vi "fp display engine resonance.vi"(7 "channel data in":sgl[][][](array[numeric]), 10 "Image Refs In":T1[](array[typedef]), 11 "DisplayRefsIn(generic class)":refnum<vi>[](array[refnum])) -> ()   [LabVIEW 2012]
uses:
  <vilib>/vision/Image Controls.llb/IMAQ Image.ctl
  Custom Controls/Ch selector.ctl
  GFG/GFGfpRefGet.vi
  GFG/GFGbooleanGet.vi
  Custom Controls/MAIN Image panel tab Control type def.ctl
  <vilib>/vision/NI_Vision_Development_Module.lvlib
  GFG/GFG library.lvlib
panel:
  in  "ROI colors":u32[](array[colorbox])=[6618880, 16716362, 16860, 16776793, 16750848, 16448250, 16716530, 9567230, 16764108, 7340212, 32639, 0, 13816530, 8421376, 8421631, 7171459, 6618880, 16716362, 16860, 16776793, 16750848, 16448250, 16716530, 9567230, 16764108, 7340212, 32639, 0, 13816530, 8421376, 8421631, 7171459, 6618880, 16716362, 16860, 16776793, 16750848, 16448250, 16716530, 9567230, 16764108, 7340212, 32639, 0, 13816530, 8421376, 8421631, 7171459, 6618880, 16716362, 16860, 16776793, 16750848, 16448250, 16716530, 9567230, 16764108, 7340212, 32639, 0, 13816530, 8421376, 8421631, 7171459, 6618880, 16716362, 16860, 16776793, 16750848, 16448250, 16716530, 9567230, 16764108, 7340212, 32639, 0, 13816530, 8421376, 8421631, 7171459, 6618880, 16716362, 16860, 16776793, 16750848, 16448250, 16716530, 9567230, 16764108, 7340212, 32639, 0, 13816530, 8421376, 8421631, 7171459, 6618880, 16716362, 16860, 16776793, 16750848, 16448250, 16716530, 9567230, 16764108, 7340212, 32639, 0, 13816530, 8421376, 8421631, 7171459, 6618880, 16716362, 16860, 16776793, 16750848, 16448250, 16716530, 9567230, 16764108, 7340212, 32639, 0, 13816530, 8421376, 8421631, 7171459, 6618880, 16716362, 16860, 16776793, 16750848, 16448250, 16716530, 9567230, 16764108, 7340212, 32639, 0, 13816530, 8421376, 8421631, 7171459, 6618880, 16716362, 16860, 16776793, 16750848, 16448250, 16716530, 9567230, 16764108, 7340212, 32639, 0, 13816530, 8421376, 8421631, 7171459, 6618880, 16716362, 16860, 16776793, 16750848, 16448250, 16716530, 9567230, 16764108, 7340212, 32639, 0, 13816530, 8421376, 8421631, 7171459, 6618880, 16716362, 16860, 16776793, 16750848, 16448250, 16716530, 9567230, 16764108, 7340212, 32639, 0, 13816530, 8421376, 8421631, 7171459, 6618880, 16716362, 16860, 16776793, 16750848, 16448250, 16716530, 9567230, 16764108, 7340212, 32639, 0, 13816530, 8421376, 8421631, 7171459, 6618880, 16716362, 16860, 16776793, 16750848, 16448250, 16716530, 9567230, 16764108, 7340212, 32639, 0, 13816530, 8421376, 8421631, 7171459, 6618880, 16716362, 16860, 16776793, 16750848, 16448250, 16716530, 9567230, 16764108, 7340212, 32639, 0, 13816530, 8421376, 8421631, 7171459, 6618880, 16716362, 16860, 16776793, 16750848, 16448250, 16716530, 9567230, 16764108, 7340212, 32639, 0, 13816530, 8421376, 8421631, 7171459, 6618880, 16716362, 16860, 16776793, 16750848, 16448250, 16716530, 9567230, 16764108, 7340212, 32639, 0, 13816530, 8421376, 8421631, 7171459, 6618880, 16716362, 16860, 16776793, 16750848, 16448250, 16716530, 9567230, 16764108, 7340212, 32639, 0, 13816530, 8421376, 8421631, 7171459, 6618880, 16716362, 16860, 16776793, 16750848, 16448250, 16716530, 9567230, 16764108, 7340212, 32639, 0, 13816530, 8421376, 8421631, 7171459, 6618880, 16716362, 16860, 16776793, 16750848, 16448250, 16716530, 9567230, 16764108, 7340212, 32639, 0, 13816530, 8421376, 8421631, 7171459, 6618880, 16716362, 16860, 16776793, 16750848, 16448250, 16716530, 9567230, 16764108, 7340212, 32639, 0, 13816530, 8421376, 8421631, 7171459, 6618880, 16716362, 16860, 16776793, 16750848, 16448250, 16716530, 9567230, 16764108, 7340212, 32639, 0, 13816530, 8421376, 8421631, 7171459, 6618880, 16716362, 16860, 16776793, 16750848, 16448250, 16716530, 9567230, 16764108, 7340212, 32639, 0, 13816530, 8421376, 8421631, 7171459, 6618880, 16716362, 16860, 16776793, 16750848, 16448250, 16716530, 9567230, 16764108, 7340212, 32639, 0, 13816530, 8421376, 8421631, 7171459, 6618880, 16716362, 16860, 16776793, 16750848, 16448250, 16716530, 9567230, 16764108, 7340212, 32639, 0, 13816530, 8421376, 8421631, 7171459]
  out "error out":errorcluster
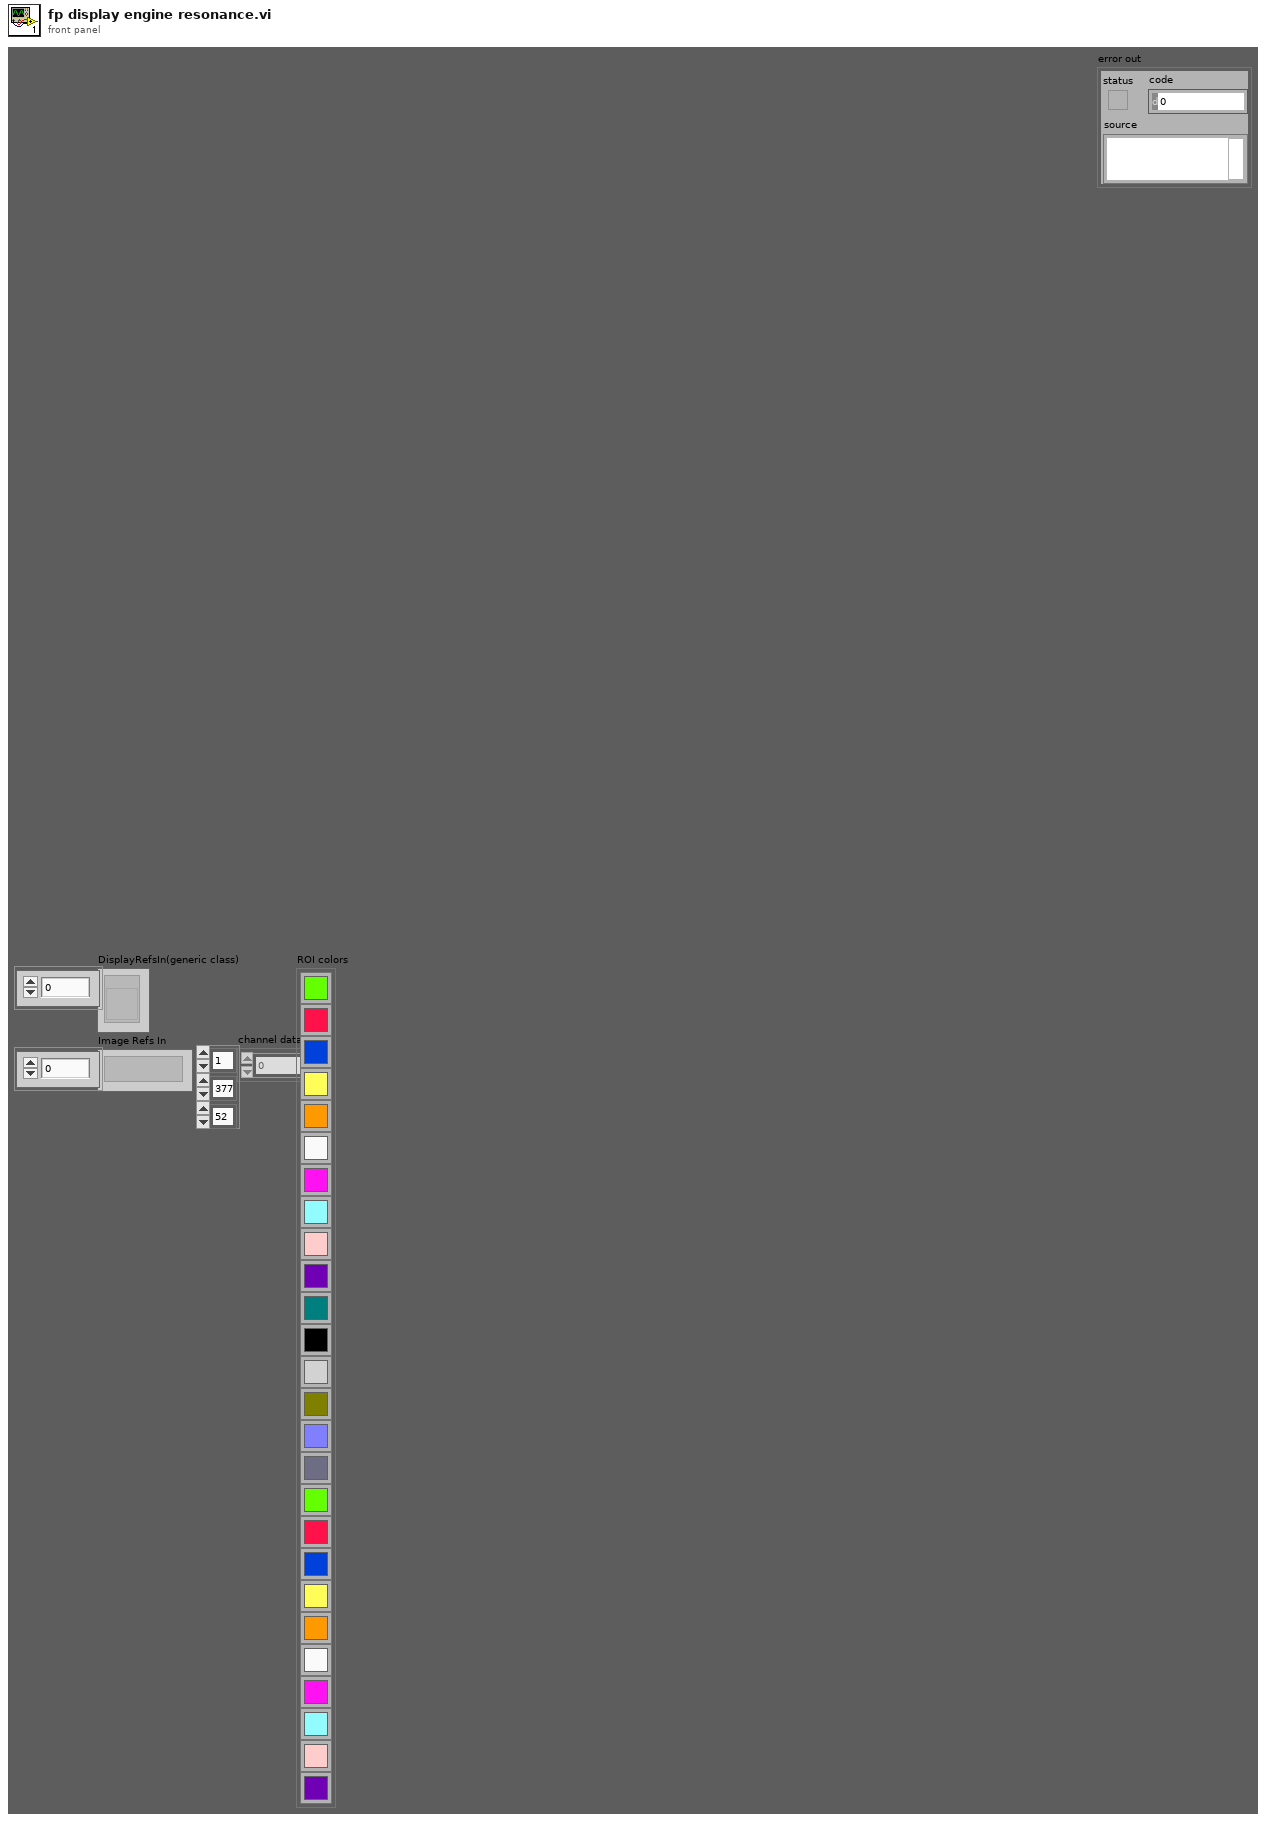
[diagram p1: front panel]
types:
  T1 = typedef "IMAQ Image.ctl" = refnum<image>
  T2 = typedef "MAIN Image panel tab Control type def.ctl" = enum32{"Channel 1", "Channel 2", "Channel 3", "Channel 4", "all channels", "RGB overlay", "ROI", "arbitrary line scan"}
  T3 = enum32{"Channel 1", "Channel 2", "Channel 3", "Channel 4", "Channel 5", "all channels", "RGB overlay", "ROI", "arbitrary line scan"}
  T4 = typedef "Ch selector.ctl" = enum16{"none", "Ch 1", "Ch 2", "Ch 3", "Ch 4", "Ch 5"}
  T5 = typedef "Image Type" = u32
  T6 = cluster{"Global Rectangle":i32[], "Contours":cluster{"Contour Type":u32, "ROI Type":u32, "Points":i32[]}[]}
  T7 = typedef "ROI Descriptor" = cluster{"Global Rectangle":i32[], "Contours":cluster{"ID":enum32{"External", "Internal"}, "Type":u32, "Coordinates":i32[]}[]}
  T8 = cluster{"WaveformChartRef":refnum<vi>, "DigitalRef":refnum<vi>, "ArrayRef":refnum<vi>, "TabControlRef":refnum<vi>, "EnumRef":refnum<vi>, "RingRef":refnum<vi>, "BooleanRef":refnum<vi>, "KnobRef":refnum<vi>, "SlideRef":refnum<vi>, "PathRef":refnum<vi>, "StringRef":refnum<vi>, "ComboBox":refnum<vi>, "WaveformGraphRef":refnum<vi>}
  T9 = cluster{"Mean Value":sgl, "Standard Variation":sgl, "Minimal Value":sgl, "Maximal Value":sgl, "Area (calibrated)":sgl, "Area (pixels)":i32, "%":sgl}[]
  T10 = cluster{"Mean Value":sgl, "Standard Variation":sgl, "Minimal Value":sgl, "Maximal Value":sgl, "Area (calibrated)":sgl, "Area (pixels)":i32, "%":sgl}
  T11 = cluster{"Contour Type":u32, "ROI Type":u32, "Points":i32[]}[]
  T12 = cluster{"Starting Value":sgl, "Incremental Value":sgl, "Histogram":u32[]}
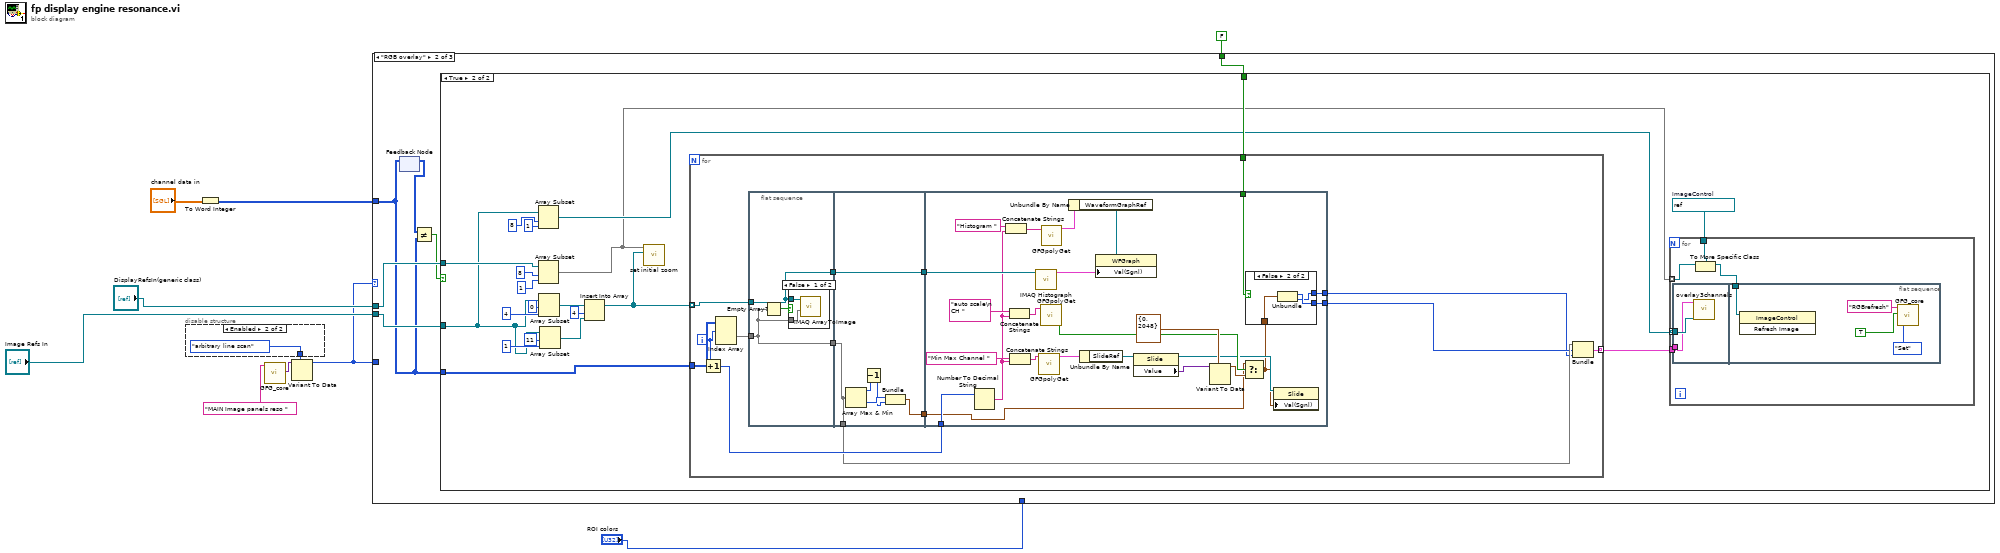
[diagram p0: block diagram]
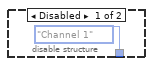
[diagram p2: hidden frame]
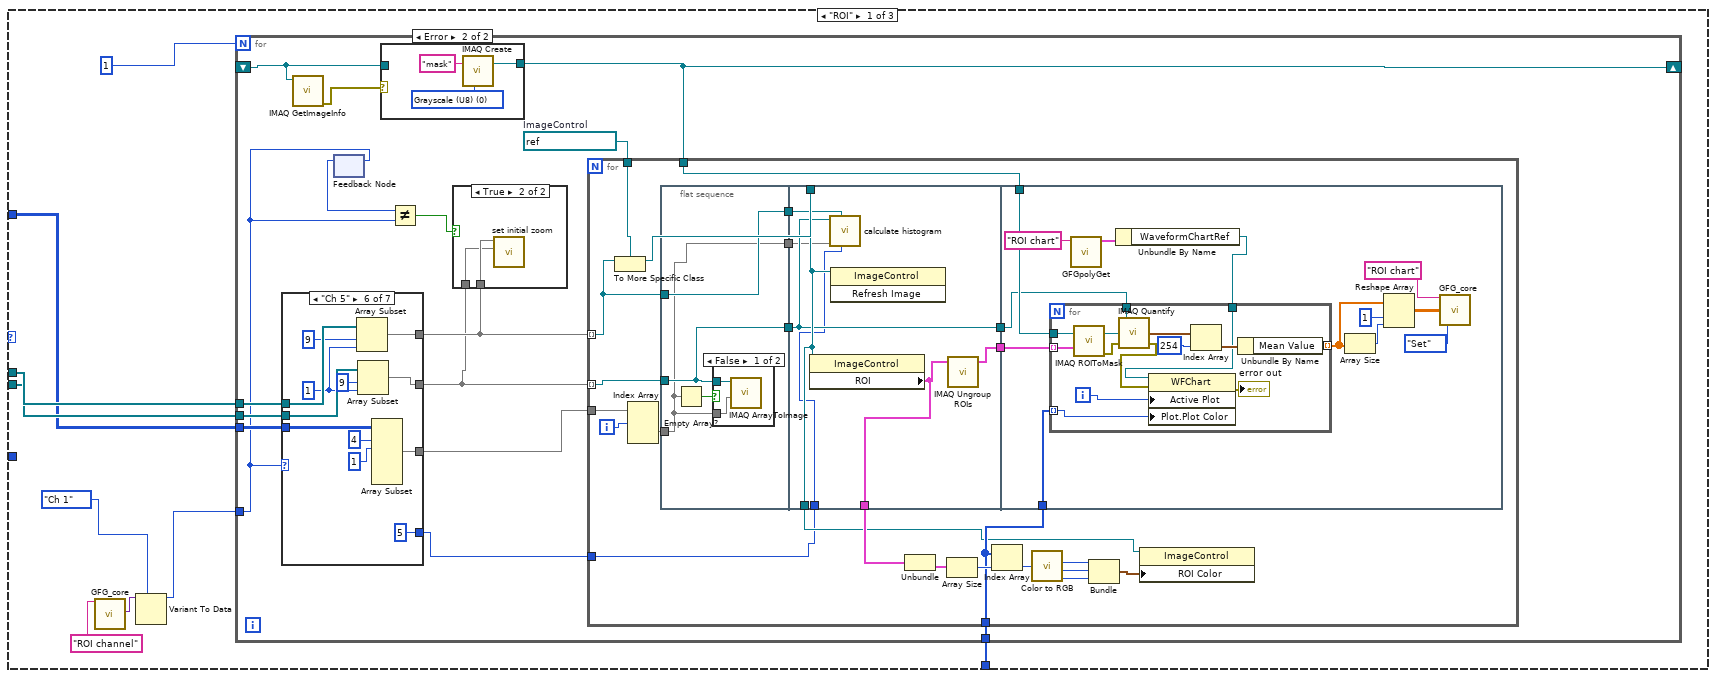
[diagram p3: hidden frame]
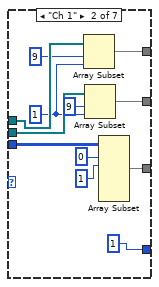
[diagram p7: hidden frame]
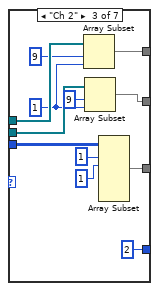
[diagram p8: hidden frame]
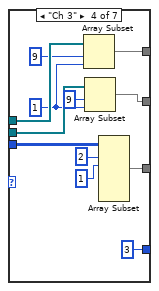
[diagram p9: hidden frame]
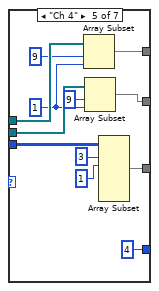
[diagram p10: hidden frame]
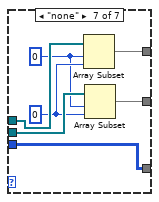
[diagram p11: hidden frame]
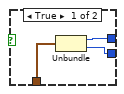
[diagram p15: hidden frame]
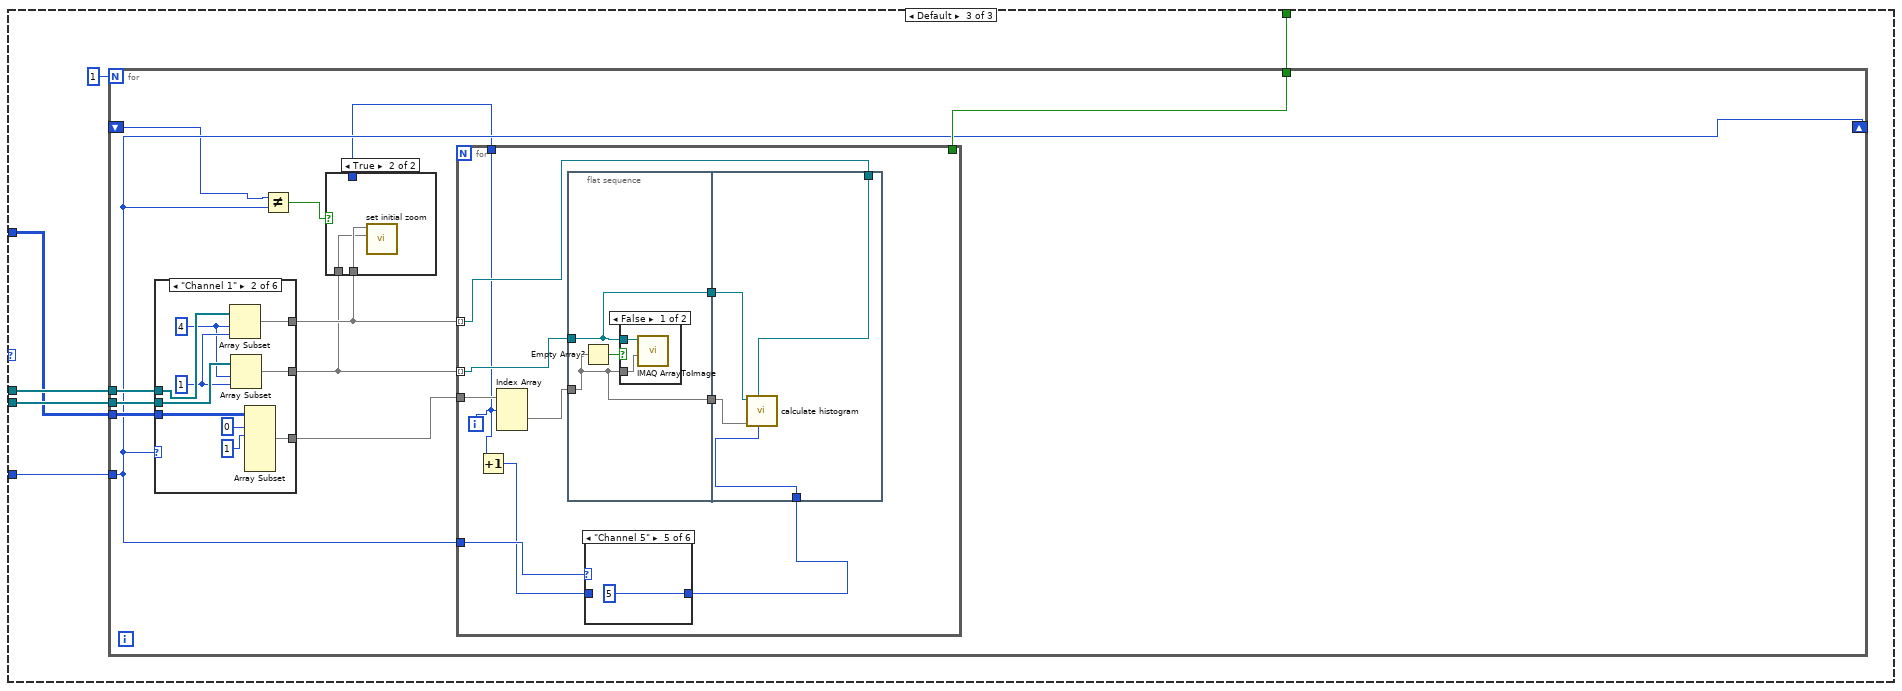
[diagram p16: hidden frame]
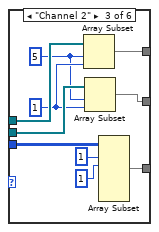
[diagram p19: hidden frame]
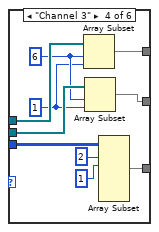
[diagram p20: hidden frame]
diagram:
  n1 = disable-structure shown="Enabled" {
    disable-tunnel: [MAIN_Image_panel_tab_Control_type_def."Channel 1" ("MAIN Image panels") T3."arbitrary line scan" ("MAIN Image panels")] -> w8
    frame Disabled {
    }
    frame Enabled {
    }
  }
  n2 = To Word Integer(number="channel data in") -> (16bit integer=w3:i16[][][])
  n3 = call "GFG_core.vi"("Variable Name in"="MAIN Image panels reso ") -> ("Variant Out"=w10:variant)  [unwired: 12 in, 6 out]
  n4 = Variant To Data(type=w8, Variant=w10) -> (data=w4:T3)  [unwired: 1 in, 1 out]
  n5 = case shown="\"RGB overlay\"" w4 {
    tunnel: w4 -> [_ _ w268]
    tunnel: "DisplayRefsIn(generic class)" -> [w20 w179 w271]
    tunnel: "Image Refs In" -> [w19 w177 w270]
    tunnel: w3 -> [w18 w175 w269]
    tunnel: FALSE -> [_ w178 w266]
    tunnel: "ROI colors" -> [w14 _ _]
    frame "ROI" {
      n6 = call "GFG_core.vi"("Variable Name in"="ROI channel") -> ("Variant Out"=w16:variant)  [unwired: 12 in, 6 out]
      n7 = Variant To Data(type=Ch_selector."Ch 1" ("ROI channel"), Variant=w16) -> (data=w15:T4)  [unwired: 1 in, 1 out]
      n8 = for {
        N: 1 -> [_]
        tunnel: w20 -> [w35]
        tunnel: w19 -> [w34]
        tunnel: w18 -> [w33]
        tunnel: w15 -> [w30]
        shift-right: [w27] -> _
        shift-left: _ -> [w26]
        tunnel: w14 -> [w24]
        w32 = refnum<vi> refnum  # ImageControl
        n9 = case shown="\"Ch 5\"" w30 {
          tunnel: w35 -> [_ w53 w65 w77 w89 w101 w108]
          tunnel: w34 -> [_ w54 w66 w78 w90 w102 w109]
          tunnel: [_ w50 w62 w74 w86 w98 w105] -> w22
          tunnel: [_ w49 w61 w73 w85 w97 w104] -> w29
          tunnel: w33 -> [_ w48 w58 w70 w82 w94 w103]
          tunnel: [_ w45 w57 w69 w81 w93 w103] -> w36
          tunnel: [_ 1 ("length") 2 ("length") 3 ("length") 4 ("length") 5 ("length") _] -> w23
          frame Default {
          }
          frame "Ch 1" {
            w52 = 1 ("length")
            n10 = Array Subset(array=w53, index=9, length=w52) -> (w49:refnum<vi>[])
            n11 = Array Subset(array=w54, index=9, length=w52) -> (w50:T1[])
            n12 = Array Subset(array=w48, index (dim 0)=0 ("index"), length (dim 0)=1 ("length")) -> (w45:i16[][][])  [unwired: 4 in]
          }
          frame "Ch 2" {
            w64 = 1 ("length")
            n13 = Array Subset(array=w65, index=9, length=w64) -> (w61:refnum<vi>[])
            n14 = Array Subset(array=w66, index=9, length=w64) -> (w62:T1[])
            n15 = Array Subset(array=w58, index (dim 0)=1 ("index"), length (dim 0)=1 ("length")) -> (w57:i16[][][])  [unwired: 4 in]
          }
          frame "Ch 3" {
            w75 = 1 ("index")
            n16 = Array Subset(array=w77, index=9, length=w75) -> (w73:refnum<vi>[])
            n17 = Array Subset(array=w78, index=9, length=w75) -> (w74:T1[])
            n18 = Array Subset(array=w70, index (dim 0)=2 ("index"), length (dim 0)=1 ("length")) -> (w69:i16[][][])  [unwired: 4 in]
          }
          frame "Ch 4" {
            w88 = 1 ("index")
            n19 = Array Subset(array=w89, index=9, length=w88) -> (w85:refnum<vi>[])
            n20 = Array Subset(array=w90, index=9, length=w88) -> (w86:T1[])
            n21 = Array Subset(array=w82, index (dim 0)=3 ("index"), length (dim 0)=1 ("length")) -> (w81:i16[][][])  [unwired: 4 in]
          }
          frame "Ch 5" {
            w100 = 1 ("index")
            n22 = Array Subset(array=w101, index=9, length=w100) -> (w97:refnum<vi>[])
            n23 = Array Subset(array=w102, index=9, length=w100) -> (w98:T1[])
            n24 = Array Subset(array=w94, index (dim 0)=4 ("index"), length (dim 0)=1 ("length")) -> (w93:i16[][][])  [unwired: 4 in]
          }
          frame "none" {
            w106 = 0 ("index")
            w107 = 0 ("length")
            n25 = Array Subset(array=w108, index=w106, length=w107) -> (w104:refnum<vi>[])
            n26 = Array Subset(array=w109, index=w106, length=w107) -> (w105:T1[])
          }
        }
        n27 = call "IMAQ GetImageInfo"("Image"=w26) -> ("error out"=w25:errorcluster)  [unwired: 3 in, 7 out]
        n28 = feedback-in #1(w30) -> ()
        n29 = feedback #1() -> (w31:T4)  [unwired: 1 in]
        n30 = case shown="Error" w25 {
          tunnel: [w37 w38] -> w27
          tunnel: w26 -> [w37 _]
          frame No Error {
          }
          frame Error {
            w39 = T5 0 items=["Grayscale (U8)", "Grayscale (I16)", "Grayscale (SGL)", "Complex (CSG)", "RGB (U32)", "HSL (U32)", "RGB (U64)"] ("Image Type")
            n31 = call "IMAQ Create"("Image Name"="mask", "Image Type"=w39) -> ("New Image"=w38:T1)  [unwired: 3 in, 1 out]
          }
        }
        n32 = Not Equal?(x=w31, y=w30) -> (x != y?=w28:bool)
        n33 = case shown="True" w28 {
          tunnel: w29 -> [_ w42]
          tunnel: w22 -> [_ w41]
          frame False {
          }
          frame True {
            n34 = call "set initial zoom.vi"("Image Refs In"=w41, "DisplayRefsIn(generic class)"=w42) -> ()  [unwired: 10 in]
          }
        }
        n35 = for {
          tunnel: w29 -> [w112] mode=indexing
          tunnel: w22 -> [w131] mode=indexing
          tunnel: w36 -> [w133]
          tunnel: w32 -> [w130]
          tunnel: w27 -> [w115]
          tunnel: w24 -> [w118]
          tunnel: w23 -> [w110]
          i -> [w128]
          n36 = To More Specific Class(target class=w130, reference=w112) -> (specific class reference=w129:refnum<vi>)  [unwired: 1 in, 1 out]
          n37 = Index Array(array=w133, index (dim 0)=w128) -> (element=w132:i16[][])  [unwired: 2 in]
          n38 = flat-sequence {
            tunnel: w132 -> [w134]
            tunnel: w131 -> [w136]
            tunnel: [w136] -> w116
            tunnel: [w135] -> w113
            tunnel: w112 -> [w135]
            tunnel: [w134] -> w111
            tunnel: w129 -> [w144]
            tunnel: [w146] -> w121
            tunnel: [w145] -> w119
            tunnel: [w142] -> w117
            tunnel: w116 -> [w142]
            tunnel: [w144] -> w114
            tunnel: w113 -> [w143]
            tunnel: w111 -> [w141]
            tunnel: w110 -> [w140]
            tunnel: w119 -> [w156]
            tunnel: w118 -> [w155]
            tunnel: w117 -> [w147]
            tunnel: w115 -> [w148]
            frame #0 {
              n39 = Empty Array?(array=w134) -> (empty?=w137:bool)
              n40 = case shown="False" w137 {
                tunnel: w136 -> [w139 _]
                tunnel: w134 -> [w138 _]
                frame False {
                  n41 = call "IMAQ ArrayToImage"("Image Pixels (I16)"=w138, "Image"=w139) -> ()  [unwired: 8 in, 2 out]
                }
                frame True {
                }
              }
            }
            frame #1 {
              n42 = property class="ImageControl"(reference=w144) -> ("ROI"=w146:T6)  [unwired: 1 in, 2 out]
              n43 = call "calculate histogram.vi"("channel no."=w140, "Image Ctrl Ref (as generic class)"=w143, "Image Array"=w141, "Image"=w142) -> ()  [unwired: 8 in]
              n44 = invoke class="ImageControl" method="Refresh Image"(reference=w144) -> ()  [unwired: 2 in, 3 out]
              n45 = call "IMAQ Ungroup ROIs"("ROI Descriptor"=w146) -> ("ROI Descriptors out"=w145:T7[])  [unwired: 3 in, 1 out]
            }
            frame #2 {
              n46 = call-poly "GFGpolyGet.vi"("Variable Name in"="ROI chart") -> ("output cluster"=w150:T8)  [unwired: 9 in, 1 out]
              n47 = Unbundle By Name(w150) -> ("WaveformChartRef"=w149:refnum<vi>)
              n48 = for {
                tunnel: w147 -> [w173]
                tunnel: w156 -> [w167] mode=indexing
                tunnel: [w169] -> w159 mode=indexing
                tunnel: w148 -> [w166]
                tunnel: w155 -> [w163] mode=indexing
                tunnel: w149 -> [w162]
                i -> [w164]
                n49 = call "IMAQ ROIToMask"("ROI Descriptor"=w167, "Image"=w166) -> ("error out"=w161:errorcluster, "Image Out"=w168:T1)  [unwired: 4 in, 1 out]
                n50 = call "IMAQ Quantify"("error in (no error)"=w161, "Image Mask"=w168, "Image"=w173) -> ("error out"=w160:errorcluster, "Region Reports"=w172:T9)  [unwired: 1 out]
                n51 = property on="Property Node" class="WFChart"(reference=w162, error in=w160, "Active Plot"=w164, "Plot.Plot Color"=w163) -> (error out=→"error out":errorcluster)  [unwired: 1 out]
                n52 = Index Array(array=w172, index=254) -> (element=w170:T10)
                n53 = Unbundle By Name(w170) -> ("Mean Value"=w169:sgl)
              }
              n54 = Array Size(array=w159) -> (size(s)=w158:i32)
              n55 = Reshape Array(w159, 1 ("dimension size"), w158) -> (w153:sgl[][])
              n56 = call "GFG_core.vi"("Variable Name in"="ROI chart", "Variant in"=w153, "Action"=enum16{"Init", "Set", "Get"}."Set") -> ()  [unwired: 10 in, 7 out]
            }
          }
          n57 = Unbundle(w121) -> ("Contours"=w126:T11)  [unwired: 1 out]
          n58 = Array Size(array=w126) -> (size(s)=w127:i32)
          n59 = Index Array(array=w118, index=w127) -> (element=w122:u32)
          n60 = call <vilib>:"Color to RGB.vi"("Color"=w122) -> ("R"=w123:u8, "G"=w124:u8, "B"=w125:u8)  [unwired: 1 out]
          n61 = Bundle("R"=w123, "G"=w124, "B"=w125) -> (w120:cluster{"R":u8, "G":u8, "B":u8})  [unwired: 1 in]
          n62 = property class="ImageControl"(reference=w114, "ROI Color"=w120) -> ()  [unwired: 1 in, 2 out]
        }
      }
    }
    frame "RGB overlay" {
      n63 = feedback-in #2(w175) -> ()
      n64 = feedback #2() -> (w176:i16[][][])  [unwired: 1 in]
      n65 = Not Equal?(x=w176, y=w175) -> (x != y?=w174:bool)
      n66 = case shown="True" w174 {
        tunnel: w179 -> [_ w199]
        tunnel: w175 -> [_ w198]
        tunnel: w178 -> [_ w197]
        tunnel: w177 -> [_ w183]
        frame False {
        }
        frame True {
          w186 = refnum<vi> refnum  # ImageControl
          n67 = Array Subset(array=w183, index=8, length=1) -> (w190:T1[])
          n68 = Array Subset(array=w199, index=8, length=1) -> (w187:refnum<vi>[])
          n69 = Array Subset(array=w183, index=0, length=4) -> (w188:T1[])
          n70 = Array Subset(array=w183, index=11, length=1) -> (w180:T1[])
          n71 = Insert Into Array(array=w188, index=4, new element=w180) -> (w182:T1[])
          n72 = call "set initial zoom.vi"("Image Refs In"=w182, "DisplayRefsIn(generic class)"=w187) -> ()  [unwired: 10 in]
          n73 = for {
            tunnel: w182 -> [w222] mode=indexing
            tunnel: w198 -> [w224]
            tunnel: w197 -> [w215]
            tunnel: [w211] -> w189 mode=indexing
            i -> [w219]
            n74 = Increment(x=w219) -> (x+1=w217:i32)
            n75 = Index Array(array=w224, index (dim 0)=w219) -> (element=w223:i16[][])  [unwired: 2 in]
            n76 = flat-sequence {
              tunnel: w223 -> [w225]
              tunnel: w222 -> [w226]
              tunnel: [w226] -> w220
              tunnel: [w225] -> w218
              tunnel: [w235] -> w221
              tunnel: w220 -> [w235]
              tunnel: w218 -> [w230]
              tunnel: [w233] -> w216
              tunnel: [w230] -> w214
              tunnel: w221 -> [w254]
              tunnel: w217 -> [w253]
              tunnel: w216 -> [w241]
              tunnel: w215 -> [w236]
              tunnel: [w238] -> w212
              tunnel: [w237] -> w213
              frame #0 {
                n77 = Empty Array?(array=w225) -> (empty?=w227:bool)
                n78 = case shown="False" w227 {
                  tunnel: w226 -> [w229 _]
                  tunnel: w225 -> [w228 _]
                  frame False {
                    n79 = call "IMAQ ArrayToImage"("Image Pixels (I16)"=w228, "Image"=w229) -> ()  [unwired: 8 in, 2 out]
                  }
                  frame True {
                  }
                }
              }
              frame #1 {
                n80 = Array Max & Min(array=w230) -> (max value=w234:i16, min value=w232:i16)  [unwired: 2 out]
                n81 = Decrement(x=w234) -> (x-1=w231:i16)
                n82 = Bundle(w232, w231) -> (w233:cluster{i16, i16})  [unwired: 1 in]
              }
              frame #2 {
                n83 = Number To Decimal String(number=w253) -> (decimal integer string=w248:string)  [unwired: 1 in]
                n84 = Concatenate Strings("Histogram " ("string"), w248) -> (w256:string)
                n85 = Concatenate Strings("auto scale\n      CH " ("Variable Name in"), w248) -> (w251:string)
                n86 = Concatenate Strings("Min Max Channel " ("Variable Name in"), w248) -> (w239:string)
                n87 = call "IMAQ Histograph"("Image"=w254) -> ("Histogram Graph"=w259:T12)  [unwired: 7 in, 3 out]
                n88 = call-poly "GFGpolyGet.vi"("Variable Name in"=w239) -> ("output cluster"=w250:T8)  [unwired: 9 in, 1 out]
                n89 = call-poly "GFGpolyGet.vi"("Variable Name in"=w251) -> ("Boolean"=w244:bool)  [unwired: 10 in]
                n90 = call-poly "GFGpolyGet.vi"("Variable Name in"=w256) -> ("output cluster"=w257:T8)  [unwired: 9 in, 1 out]
                n91 = Unbundle By Name(w257) -> ("WaveformGraphRef"=w258:refnum<vi>)
                n92 = Unbundle By Name(w250) -> ("SlideRef"=w247:refnum<vi>)
                n93 = property class="WFGraph"(reference=w258, "Val(Sgnl)"=w259) -> ()  [unwired: 1 in, 2 out]
                n94 = property class="Slide"(reference=w247) -> (reference out=w242:refnum<vi>, "Value"=w246:variant)  [unwired: 1 in, 1 out]
                n95 = Variant To Data(type=cluster{i32, i32} {0, 2048} ("channel1"), Variant=w246) -> (data=w243:cluster{i32, i32})  [unwired: 1 in, 1 out]
                n96 = Select(t=w241, s=w244, f=w243) -> (s? t:f=w240:cluster{i32, i32})
                n97 = case shown="False" w236 {
                  tunnel: w240 -> [w262 w265]
                  tunnel: [w261 w263] -> w238
                  tunnel: [w260 w264] -> w237
                  frame True {
                    n98 = Unbundle(w262) -> (w261:i32, w260:i32)
                  }
                  frame False {
                    n99 = Unbundle(w265) -> (w264:i32, w263:i32)
                  }
                }
                n100 = property class="Slide"(reference=w242, "Val(Sgnl)"=w240) -> ()  [unwired: 1 in, 2 out]
              }
            }
            n101 = Bundle(w214, w213, w212) -> (w211:cluster{i16[][], i32, i32})  [unwired: 1 in]
          }
          n102 = for {
            tunnel: w190 -> [w204] mode=indexing
            tunnel: w189 -> [w203]
            tunnel: w187 -> [w202] mode=indexing
            tunnel: w186 -> [w201]
            n103 = flat-sequence {
              tunnel: w204 -> [w206]
              tunnel: w203 -> [w205]
              tunnel: w200 -> [w210]
              frame #0 {
                n104 = call "overlay3channels.vi"("RGB Overlay"=w206, "Array"=w205) -> ()  [unwired: 10 in]
              }
              frame #1 {
                n105 = invoke class="ImageControl" method="Refresh Image"(reference=w210) -> ()  [unwired: 2 in, 3 out]
                n106 = call "GFG_core.vi"("Variable Name in"="RGBrefresh", "Variant in"=TRUE, "Action"=enum16{"Init", "Set", "Get"}."Set") -> ()  [unwired: 10 in, 7 out]
              }
            }
            n107 = To More Specific Class(target class=w201, reference=w202) -> (specific class reference=w200:refnum<vi>)  [unwired: 1 in, 1 out]
          }
        }
      }
    }
    frame Default {
      n108 = for {
        N: 1 -> [_]
        tunnel: w271 -> [w281]
        tunnel: w270 -> [w280]
        tunnel: w269 -> [w279]
        tunnel: w268 -> [w274]
        tunnel: w266 -> [w276]
        shift-right: [w274] -> _
        shift-left: _ -> [w273]
        n109 = case shown="\"Channel 1\"" w274 {
          tunnel: w281 -> [_ w293 w303 w313 w323 w333]
          tunnel: w280 -> [_ w294 w304 w314 w324 w334]
          tunnel: [_ w290 w300 w310 w320 w330] -> w275
          tunnel: [_ w289 w299 w309 w319 w329] -> w278
          tunnel: w279 -> [_ w288 w296 w306 w316 w326]
          tunnel: [_ w285 w295 w305 w315 w325] -> w282
          frame Default {
          }
          frame "Channel 1" {
            w291 = 4 ("index")
            w292 = 1 ("length")
            n110 = Array Subset(array=w293, index=w291, length=w292) -> (w289:refnum<vi>[])
            n111 = Array Subset(array=w294, index=w291, length=w292) -> (w290:T1[])
            n112 = Array Subset(array=w288, index (dim 0)=0 ("index"), length (dim 0)=1 ("length")) -> (w285:i16[][][])  [unwired: 4 in]
          }
          frame "Channel 2" {
            w301 = 5 ("index")
            w302 = 1 ("length")
            n113 = Array Subset(array=w303, index=w301, length=w302) -> (w299:refnum<vi>[])
            n114 = Array Subset(array=w304, index=w301, length=w302) -> (w300:T1[])
            n115 = Array Subset(array=w296, index (dim 0)=1 ("index"), length (dim 0)=1 ("length")) -> (w295:i16[][][])  [unwired: 4 in]
          }
          frame "Channel 3" {
            w311 = 1 ("index")
            w312 = 6 ("index")
            n116 = Array Subset(array=w313, index=w312, length=w311) -> (w309:refnum<vi>[])
            n117 = Array Subset(array=w314, index=w312, length=w311) -> (w310:T1[])
            n118 = Array Subset(array=w306, index (dim 0)=2 ("index"), length (dim 0)=1 ("length")) -> (w305:i16[][][])  [unwired: 4 in]
          }
          frame "Channel 4" {
            w321 = 7 ("index")
            w322 = 1 ("index")
            n119 = Array Subset(array=w323, index=w321, length=w322) -> (w319:refnum<vi>[])
            n120 = Array Subset(array=w324, index=w321, length=w322) -> (w320:T1[])
            n121 = Array Subset(array=w316, index (dim 0)=3 ("index"), length (dim 0)=1 ("length")) -> (w315:i16[][][])  [unwired: 4 in]
          }
          frame "Channel 5" {
            w331 = 11 ("index")
            w332 = 1 ("index")
            n122 = Array Subset(array=w333, index=w331, length=w332) -> (w329:refnum<vi>[])
            n123 = Array Subset(array=w334, index=w331, length=w332) -> (w330:T1[])
            n124 = Array Subset(array=w326, index (dim 0)=4 ("index"), length (dim 0)=1 ("length")) -> (w325:i16[][][])  [unwired: 4 in]
          }
        }
        n125 = Not Equal?(x=w273, y=w274) -> (x != y?=w277:bool)
        n126 = for {
          tunnel: w278 -> [w337] mode=indexing
          tunnel: w275 -> [w339] mode=indexing
          tunnel: w282 -> [w344]
          tunnel: w274 -> [w343]
          tunnel: w276 -> [_]
          tunnel: [w336] -> w272
          i -> [w336]
          n127 = Increment(x=w336) -> (x+1=w342:i32)
          n128 = Index Array(array=w344, index (dim 0)=w336) -> (element=w335:i16[][])  [unwired: 2 in]
          n129 = flat-sequence {
            tunnel: w335 -> [w345]
            tunnel: w339 -> [w346]
            tunnel: [w346] -> w341
            tunnel: [w345] -> w340
            tunnel: w341 -> [w351]
            tunnel: w340 -> [w353]
            tunnel: w338 -> [w352]
            tunnel: w337 -> [w350]
            frame #0 {
              n130 = Empty Array?(array=w345) -> (empty?=w347:bool)
              n131 = case shown="False" w347 {
                tunnel: w346 -> [w349 _]
                tunnel: w345 -> [w348 _]
                frame False {
                  n132 = call "IMAQ ArrayToImage"("Image Pixels (I16)"=w348, "Image"=w349) -> ()  [unwired: 8 in, 2 out]
                }
                frame True {
                }
              }
            }
            frame #1 {
              n133 = call "calculate histogram.vi"("channel no."=w352, "Image Ctrl Ref (as generic class)"=w350, "Image Array"=w353, "Image"=w351) -> ()  [unwired: 8 in]
            }
          }
          n134 = case shown="\"Channel 5\"" w343 {
            tunnel: [1 2 3 4 5 w359] -> w338
            tunnel: w342 -> [_ _ _ _ _ w359]
            frame "Channel 1", Default {
            }
            frame "Channel 2" {
            }
            frame "Channel 3" {
            }
            frame "Channel 4" {
            }
            frame "Channel 5" {
            }
            frame "all channels" {
            }
          }
        }
        n135 = case shown="True" w277 {
          tunnel: w278 -> [_ w284]
          tunnel: w275 -> [_ w283]
          tunnel: w272 -> [_ _]
          frame False {
          }
          frame True {
            n136 = call "set initial zoom.vi"("Image Refs In"=w283, "DisplayRefsIn(generic class)"=w284) -> ()  [unwired: 10 in]
          }
        }
      }
    }
  }
